vi "FOCUS_V42_H37.vi"(9 "X-pixels":sgl=256.0, 11 "Run":bool) -> (0 "Retrace pixels":sgl, 10 "Pixel Clock (Hz)":sgl)   [LabVIEW 2010] (continued)
      n95 = local write "ScanLineFScope"(sgl[][] [[0.026666667, 0.10555588, 0.18413667, 0.2620946, 0.33912018, 0.4149288, 0.48917702, 0.5616217, 0.6319491, 0.69988036, 0.7651882, 0.8275282, 0.88674605, 0.9425593, 0.9947472, 1.043162, 1.087492, 1.127687, 1.163523, 1.1948596, 1.2216425, 1.2436236, 1.2608614, 1.2732126, 1.2806307, 1.2831601, 1.280641, 1.2732344, 1.2608918, 1.2436653, 1.2216938, 1.1949208, 1.1635948, 1.1277666, 1.0875816, 1.0432596, 0.9948533, 0.9426741, 0.8868671, 0.8276569, 0.7653226, 0.70002097, 0.6320957, 0.5617722, 0.48933217, 0.41508698, 0.33928153, 0.2622585, 0.18430196, 0.10572225, 0.026833316, -0.052056268, -0.13063815, -0.20859744, -0.28562555, -0.36143658, -0.43568876, -0.50813806, -0.57846946, -0.6464066, -0.71171933, -0.77406645, -0.833292, -0.8891114, -0.941308, -0.9897297, -1.0340693, -1.0742743, -1.110118, -1.1414653, -1.1682563, -1.1902486, -1.2074977, -1.2198576, -1.2272873, -1.2298253, -1.2273177, -1.2199228, -1.2075888, -1.1903737, -1.1684103, -1.1416483, -1.110333, -1.0745125, -1.0343375, -0.99002266, -0.9416256, -0.8894551, -0.83365417, -0.7744517, -0.71212274, -0.6468276, -0.57890815, -0.5085887, -0.43615317, -0.36191097, -0.28610873, -0.20908824, -0.13062674, -0.05199747], [-1.2831608, -1.2806358, -1.2732235, -1.2608767, -1.2436445, -1.2216686, -1.1948903, -1.163559, -1.1277268, -1.0875369, -1.0432112, -0.9948003, -0.94261676, -0.88680667, -0.8275926, -0.7652557, -0.69995075, -0.6320225, -0.56169707, -0.48925468, -0.41500804, -0.33920097, -0.26217666, -0.18421942, -0.105639175, -0.026750105, 0.052139297, 0.13072063, 0.20867924, 0.28570607, 0.3615159, 0.4357661, 0.5082131, 0.57854253, 0.6464767, 0.71178705, 0.7741306, 0.83335227, 0.88916856, 0.9413609, 0.9897791, 1.034114, 1.0743139, 1.1101538, 1.1414957, 1.1682826, 1.1902695, 1.2075129, 1.2198684, 1.2272923, 1.2298261, 1.2273127, 1.2199119, 1.2075737, 1.1903529, 1.1683854, 1.1416179, 1.1102973, 1.0744729, 1.034293, 0.98997456, 0.94157284, 0.889398, 0.833594, 0.7743877, 0.7120561, 0.6467577, 0.5788353, 0.50851387, 0.4360761, 0.3618324, 0.28602856, 0.20900682, 0.13105093, 0.052471776, -0.026417017, -0.10530679, -0.18388921, -0.2618492, -0.33887854, -0.4146908, -0.48894495, -0.56139654, -0.63172984, -0.69966996, -0.76498514, -0.82733583, -0.8865652, -0.94238764, -0.9945887, -1.0430137, -1.0873581, -1.127568, -1.1634157, -1.1947683, -1.2215633, -1.2435613, -1.260816, -1.2693994, -1.2762786]] ("transposed array")) -> ()
    }
  }
  n96 = Type Cast(type="" ("name or relative path"), x=w48) -> (*(type *) &x=w45:string)
  n97 = Type Cast(type=tag "" ("6229 Device 2"), x=w65) -> (*(type *) &x=w64:tag)
  n98 = Type Cast(type=refnum<visa-resource-name> " " ("VISA Sutter MP-285"), x=w50) -> (*(type *) &x=w49:refnum<visa-resource-name>)
  n99 = Type Cast(type=refnum<visa-resource-name> refnum ("VISA Sutter MP-285"), x=w54) -> (*(type *) &x=w4:refnum<visa-resource-name>)
  n100 = property on="Run" class="Bool (strict)"("Visible"=w100) -> ()  [unwired: 2 in, 2 out]
  n101 = local write "End experiment"(w101) -> ()
  n102 = property on="colour table" class="Arr (strict)"("Value"=w37) -> ()  [unwired: 2 in, 2 out]
  n103 = property on="Galvos" class="XYGraph (strict)"("X Scale.Range:Minimum"=w3, "X Scale.Range:Maximum"="Scangraph scaling", "Y Scale.Range:Minimum"=w2, "Y Scale.Range:Maximum"="Scangraph scaling") -> ()  [unwired: 2 in, 2 out]
  n104 = Type Cast(type=u16 0 ("Program Version"), x=w84) -> (*(type *) &x=→"Program Version":u16)
  n105 = String To Path(string=w45) -> (path=w44:path)
  n106 = local write "FocusModeSelector"(TRUE ("FocusModeSelector")) -> ()
  n107 = local write "new FreeLine?"(FALSE ("new udl?")) -> ()
  n108 = local write "NewScanpattern"(FALSE ("NewScanpattern")) -> ()
  n109 = local write "VISA XPG-ADC"(w49) -> ()
  n110 = local write "AO/DIO Device"(w67) -> ()
  n111 = local write "VISA Sutter MP-285"(w4) -> ()
  n112 = property on="stop 2" class="Bool (strict)"("Visible"=w100) -> ()  [unwired: 2 in, 2 out]
  n113 = property on="Scan format" class="Ring (strict)"("Disabled"=u8 0) -> ()  [unwired: 2 in, 2 out]
  n114 = local write "AI Device"(w64) -> ()
  n115 = local write "MaiTai setting Path"(w44) -> ()
  n116 = local write "reset?"(125.0 ("reset?")) -> ()
  n117 = property on="Image 2" class="IntGraph (strict)"("Color Table"=w37) -> ()  [unwired: 2 in, 2 out]
  n118 = property on="End experiment" class="Bool (strict)"("Visible"=w100) -> ()  [unwired: 2 in, 2 out]
  n119 = local write "stop 2"(w101) -> ()
  n120 = property on="Hit Graph" class="IntGraph (strict)"("Color Table"=w37) -> ()  [unwired: 2 in, 2 out]
  n121 = while {
    tunnel: w6 -> [w207]
    tunnel: [w162] -> w5
    stop <- w163 stop-if-true
    n122 = flat-sequence {
      tunnel: [w1453] -> w295
      tunnel: w295 -> [w1668]
      tunnel: [w1626] -> w177
      tunnel: [w1641] -> w175
      tunnel: ["Zoom 1 scan voltage"] -> w174
      tunnel: [w1638] -> w173
      tunnel: [w1637] -> w172
      tunnel: [w1622] -> w170
      tunnel: [w1621] -> w169
      tunnel: [w2017] -> w259
      tunnel: [w2016] -> w288
      tunnel: [w1902] -> w290
      tunnel: [w2008] -> w260
      tunnel: [w1963] -> w298
      tunnel: [w1956] -> w262
      tunnel: [w1923] -> w297
      tunnel: [w2014] -> w261
      tunnel: [w2013] -> w285
      tunnel: [w2038] -> w283
      tunnel: [w2031] -> w282
      tunnel: w176 -> [w1887]
      tunnel: w186 -> [w1886]
      tunnel: [w1885] -> w182
      tunnel: w177 -> [w1873]
      tunnel: w175 -> [w1859]
      tunnel: w174 -> [w1872]
      tunnel: w173 -> [w1871]
      tunnel: w172 -> [w1870]
      tunnel: w171 -> [w1868]
      tunnel: w170 -> [w1864]
      tunnel: w169 -> [w1863]
      tunnel: [w1860] -> w168
      frame #0 {
        n123 = property on="Fiberscope" class="TabCtl (strict)"("Visible"="Fiberscope\nMode") -> ()  [unwired: 2 in, 2 out]
        n124 = property on="Hit Graph" class="IntGraph (strict)"("Visible"="Fiberscope\nMode") -> ()  [unwired: 2 in, 2 out]
        n125 = property on="Scale" class="Slide (strict)"("Visible"="Fiberscope\nMode") -> ()  [unwired: 2 in, 2 out]
        n126 = case shown="False" "Fiberscope\nMode" {
          tunnel: ["Mode selector" "Mode selectorFScope"] -> w1453
          frame False {
            n127 = case shown="0, Default" "Scan format" {
              tunnel: [w1559 sgl 64.0 ("X-pixels") sgl 128.0 ("X-pixels") sgl 256.0 ("X-pixels") sgl 512.0 ("X-pixels") sgl 32.0 ("X-pixels")] -> w1484
              tunnel: [w1558 sgl 64.0 ("Y-lines") sgl 128.0 ("Y-lines") sgl 256.0 ("Y-lines") sgl 512.0 ("Y-lines") sgl 32.0 ("Y-lines")] -> w1483
              tunnel: [w1557 sgl 2.0 ("line scan time (ms)") sgl 2.0 ("line scan time (ms)") sgl 2.0 ("line scan time (ms)") sgl 2.0 ("line scan time (ms)") sgl 1.0 ("line scan time (ms)")] -> w1482
              tunnel: [0 2 2 2 2 2] -> w1481
              frame 0, Default {
                n128 = local read "line scan time (ms)"() -> (w1557:sgl)
                n129 = local read "X-pixels"() -> (w1559:sgl)
                n130 = local read "Y-lines"() -> (w1558:sgl)
              }
              frame 1 {
              }
              frame 2 {
              }
              frame 3 {
              }
              frame 4 {
              }
              frame 5 {
              }
            }
            n131 = case shown="0, Default" "Mode selector" {
              tunnel: [2 0 2 2 0 2] -> w1465
              tunnel: [0 1 2 3 1 4] -> w1475
              tunnel: [w1496 w1506 0 w1527 w1537 w1547] -> w1471
              tunnel: w1481 -> [w1496 w1506 _ _ w1537 _]
              tunnel: [0 0 2 2 0 2] -> w1466
              tunnel: [w1501 w1511 u16 0 ("Scan format") u16 0 ("Scan format") w1542 u16 0 ("Scan format")] -> w1480
              tunnel: [TRUE ("Visible") FALSE ("Visible") FALSE ("Visible") FALSE ("Visible") FALSE ("Visible") FALSE ("Visible")] -> w1473
              tunnel: [u8 2 ("Disabled") u8 2 ("Disabled") u8 2 ("Disabled") u8 0 ("Disabled") u8 2 ("Disabled") u8 0 ("Disabled")] -> w1470
              tunnel: [2 2 2 2 2 0] -> w1461
              tunnel: [2 0 0 2 0 2] -> w1464
              tunnel: [w1496 w1506 2 w1527 w1537 w1547] -> w1463
              tunnel: [u8 2 ("Disabled") u8 2 ("Disabled") u8 0 ("Disabled") u8 0 ("Disabled") u8 2 ("Disabled") u8 2 ("Disabled")] -> w1462
              frame 0, Default {
                # "Focus mode"
                n132 = local read "Scan format"() -> (w1501:u16)
              }
              frame 1 {
                # "frame scan"
                n133 = local read "Scan format"() -> (w1511:u16)
              }
              frame 2 {
                # "straight line scan"
              }
              frame 3 {
                w1527 = 2
                # "user-defined line"
              }
              frame 4 {
                # "frame scan piezo"
                n134 = local read "Scan format"() -> (w1542:u16)
              }
              frame 5 {
                w1547 = 2
                # "user-defined line 3D"
              }
            }
            "frame/line indicator" <- w1475
            n135 = Less?(x=w1475, y=u16 3) -> (x < y?=w1477:bool)
            n136 = case shown="False" w1477 {
              tunnel: [TRUE ("Visible") FALSE ("Visible")] -> w1476
              tunnel: [w1488 FALSE ("Visible")] -> w1472
              frame False {
                n137 = property on="Image 3" class="IntGraph (strict)"() -> ("Visible"=w1488:bool)  [unwired: 2 in, 2 out]
              }
              frame True {
              }
            }
            n138 = case shown="3" "Scan format 2" {
              tunnel: [i16 10 ("X-pixels") i16 20 ("X-pixels") i16 40 ("X-pixels") i16 60 ("X-pixels")] -> w1468
              frame 0, Default {
              }
              frame 1 {
              }
              frame 2 {
              }
              frame 3 {
              }
            }
            n139 = local write "X-pixels"(w1484) -> ()
            n140 = local write "Y-lines"(w1483) -> ()
            n141 = local write "line scan time (ms)"(w1482) -> ()
            n142 = property on="phase shift [°]" class="DigNum (strict)"("Disabled"=w1461) -> ()  [unwired: 2 in, 2 out]
            n143 = local write "Scan format"(w1480) -> ()
            n144 = property on="Number of frames" class="DigNum (strict)"("Disabled"=w1464) -> ()  [unwired: 2 in, 2 out]
            n145 = property on="Averaging" class="DigNum (strict)"("Disabled"=w1465) -> ()  [unwired: 2 in, 2 out]
            n146 = property on="z-step (um)" class="DigNum (strict)"("Disabled"=w1465) -> ()  [unwired: 2 in, 2 out]
            n147 = property on="Scan format" class="Ring (strict)"("Disabled"=w1466) -> ()  [unwired: 2 in, 2 out]
            n148 = property on="X-pixels" class="DigNum (strict)"("Disabled"=w1471) -> ()  [unwired: 2 in, 2 out]
            n149 = property on="#" class="DigNum (strict)"("Disabled"=w1471) -> ()  [unwired: 2 in, 2 out]
            n150 = property on="line scan time (ms)" class="DigNum (strict)"("Disabled"=w1471) -> ()  [unwired: 2 in, 2 out]
            n151 = property on="#" class="DigNum (strict)"("Disabled"=w1470) -> ()  [unwired: 2 in, 2 out]
            n152 = property on="Y-lines FreeLine" class="DigNum (strict)"("Disabled"=w1470) -> ()  [unwired: 2 in, 2 out]
            n153 = property on="Y-Scale" class="Bool (strict)"("Disabled"=w1462) -> ()  [unwired: 2 in, 2 out]
            n154 = local write "ImageSelector"(w1472) -> ()
            n155 = property on="XY Graph 1" class="XYGraph (strict)"("Visible"=w1476) -> ()  [unwired: 2 in, 2 out]
            n156 = property on="XY Graph 2" class="XYGraph (strict)"("Visible"=w1476) -> ()  [unwired: 2 in, 2 out]
            n157 = property on="Image 3" class="IntGraph (strict)"("Visible"=w1472) -> ()  [unwired: 2 in, 2 out]
            n158 = property on="Histogram1" class="XYGraph (strict)"("Visible"=w1472) -> ()  [unwired: 2 in, 2 out]
            n159 = property on="Y-lines" class="DigNum (strict)"("Disabled"=w1463) -> ()  [unwired: 2 in, 2 out]
            n160 = Divide(x=4000.0, y=w1468) -> (x/y=→"pixelstoµm":dbl)
            n161 = property on="FocusModeSelector" class="Bool (strict)"("Visible"=w1473) -> ()  [unwired: 2 in, 2 out]
            n162 = property on="XY Graph 3" class="XYGraph (strict)"("Visible"=FALSE) -> ()  [unwired: 2 in, 2 out]
            n163 = property on="XY Graph 4" class="XYGraph (strict)"("Visible"=w1476) -> ()  [unwired: 2 in, 2 out]
            n164 = property on="Image 4" class="IntGraph (strict)"("Visible"=w1472) -> ()  [unwired: 2 in, 2 out]
            n165 = property on="Amplitude Factor" class="DigNum (strict)"("Disabled"=w1461) -> ()  [unwired: 2 in, 2 out]
            n166 = property on="z frequency" class="Slide (strict)"("Disabled"=w1461) -> ()  [unwired: 2 in, 2 out]
            n167 = property on="Histogram2" class="XYGraph (strict)"("Visible"=w1472) -> ()  [unwired: 2 in, 2 out]
            n168 = local write "Open?"(FALSE ("Open?")) -> ()
            n169 = property on="new FreeLine?" class="Bool (strict)"("Disabled"=w1470) -> ()  [unwired: 2 in, 2 out]
            n170 = property on="#" class="DigNum (strict)"("Disabled"=w1464) -> ()  [unwired: 2 in, 2 out]
            n171 = property on="#" class="DigNum (strict)"("Disabled"=w1465) -> ()  [unwired: 2 in, 2 out]
            n172 = property on="Time interval [s]" class="DigNum (strict)"("Disabled"=w1465) -> ()  [unwired: 2 in, 2 out]
            n173 = property on="Number of stacks" class="DigNum (strict)"("Disabled"=w1465) -> ()  [unwired: 2 in, 2 out]
            n174 = property on="#" class="DigNum (strict)"("Disabled"=w1465) -> ()  [unwired: 2 in, 2 out]
            n175 = property on="Cusp Delay" class="DigNum (strict)"("Disabled"=w1466) -> ()  [unwired: 2 in, 2 out]
          }
          frame True {
            n176 = local write "Mode selector"("Mode selectorFScope") -> ()
            n177 = case shown="0, Default" "Mode selectorFScope" {
              tunnel: [u16 2 ("Mode selectorFScope") u16 0 ("Mode selectorFScope") u16 2 ("Mode selectorFScope")] -> w1580
              tunnel: [u16 0 ("Mode selectorFScope") u16 0 ("Mode selectorFScope") u16 2 ("Mode selectorFScope")] -> w1583
              tunnel: [w1594 w1597 u16 0 ("Scan format FScope")] -> w1582
              frame 0, Default {
                n178 = local read "Scan format FScope"() -> (w1594:u16)
              }
              frame 1 {
                n179 = local read "Scan format FScope"() -> (w1597:u16)
              }
              frame 2 {
              }
            }
            n180 = local write "frame/line indicator"("Mode selectorFScope") -> ()
            n181 = local write "Time interval [s]"("Time interval [s]") -> ()
            n182 = local write "Number of stacks"("Number of Stacks") -> ()
            n183 = local read "Number of Frames"() -> (w1589:sgl)
            n184 = case shown="0, Default" "Scan format FScope" {
              tunnel: [w1605 sgl 64.0 ("X dim") sgl 128.0 ("X dim") sgl 256.0 ("X dim") sgl 512.0 ("X dim") sgl 32.0 ("X dim")] -> w1591
              tunnel: [w1604 sgl 64.0 ("Y dim") sgl 128.0 ("Y dim") sgl 256.0 ("Y dim") sgl 512.0 ("Y dim") sgl 32.0 ("Y dim")] -> w1590
              tunnel: [u8 0 ("Disabled") u8 2 ("Disabled") u8 2 ("Disabled") u8 2 ("Disabled") u8 2 ("Disabled") u8 2 ("Disabled")] -> w1592
              frame 0, Default {
                n185 = local read "Y dim"() -> (w1604:sgl)
                n186 = local read "X dim"() -> (w1605:sgl)
              }
              frame 1 {
              }
              frame 2 {
              }
              frame 3 {
              }
              frame 4 {
              }
              frame 5 {
              }
            }
            n187 = local read "Averaging"() -> (w1588:sgl)
            n188 = local write "Scan format FScope"(w1582) -> ()
            n189 = property on="Scan format FScope" class="Ring (strict)"("Disabled"=w1583) -> ()  [unwired: 2 in, 2 out]
            n190 = property on="Time interval [s]" class="DigNum (strict)"("Disabled"=w1580) -> ()  [unwired: 2 in, 2 out]
            n191 = property on="Number of Stacks" class="DigNum (strict)"("Disabled"=w1580) -> ()  [unwired: 2 in, 2 out]
            n192 = property on="Number of Frames" class="DigNum (strict)"("Disabled"=w1580) -> ()  [unwired: 2 in, 2 out]
            n193 = property on="Averaging" class="DigNum (strict)"("Disabled"=w1580) -> ()  [unwired: 2 in, 2 out]
            n194 = property on="#" class="DigNum (strict)"("Disabled"=w1580) -> ()  [unwired: 2 in, 2 out]
            n195 = property on="#" class="DigNum (strict)"("Disabled"=w1580) -> ()  [unwired: 2 in, 2 out]
            n196 = property on="#" class="DigNum (strict)"("Disabled"=w1580) -> ()  [unwired: 2 in, 2 out]
            n197 = local write "X dim"(w1591) -> ()
            n198 = local write "Y dim"(w1590) -> ()
            n199 = property on="Y dim" class="DigNum (strict)"("Disabled"=w1592) -> ()  [unwired: 2 in, 2 out]
            n200 = local write "Number of frames"(w1589) -> ()
            n201 = local write "Averaging"(w1588) -> ()
            n202 = global write "GlobelFSCOPE.vi" "X dim"(w1591) -> ()
            n203 = global write "GlobelFSCOPE.vi" "Y dim"(w1590) -> ()
            n204 = property on="X dim" class="DigNum (strict)"("Disabled"=w1592) -> ()  [unwired: 2 in, 2 out]
            n205 = local write "X-pixels"("X dim") -> ()
            n206 = local write "Y-lines"("Y dim") -> ()
            n207 = global write "GlobelFSCOPE.vi" "Y dim"("Y dim") -> ()
            n208 = global write "GlobelFSCOPE.vi" "X dim"("X dim") -> ()
          }
        }
        n209 = local read "GetFirst"() -> (w1447:bool)
        n210 = local read "GetLast"() -> (w1446:bool)
        n211 = And(x=w1447, y=w1446) -> (x .and. y?=w1445:bool)
        n212 = case shown="True" w1445 {
          frame False {
          }
          frame True {
            n213 = local read "Number of frames"() -> (w1457:sgl)
            n214 = local read "FirstPosition"() -> (w1454:sgl)
            n215 = local read "LastPosition"() -> (w1455:sgl)
            n216 = Decrement(x=w1457) -> (x-1=w1458:sgl)
            n217 = Subtract(x=w1455, y=w1454) -> (x-y=w1459:sgl)
            n218 = Divide(x=w1459, y=w1458) -> (x/y=w1456:sgl)
            n219 = local write "z-step (um)"(w1456) -> ()
          }
        }
        n220 = Get Date/Time String(date format (0)=enum16{"short", "long", "abbreviated"}."abbreviated") -> (time string=→"Time":string)  [unwired: 2 in, 1 out]
        n221 = Format Date/Time String(time format string (%c)="%m%d%y") -> (date/time string=→"Date":string)  [unwired: 2 in]
      }
      frame #1 {
        # "Line scan position and measurement cursors"
        n222 = local read "frame/line indicator"() -> (w1641:u16)
        n223 = Less?(x=w1668, y=3.0) -> (x < y?=w1663:bool)
        n224 = And(x="View line\ncheck box", y=w1663) -> (x .and. y?=w1667:bool)
        n225 = And(x=w1663, y="Measurement cursor check box") -> (x .and. y?=w1662:bool)
        n226 = control-ref of="Image 2"() -> (w1665:refnum<vi>)
        n227 = control-ref of="Image 1"() -> (w1666:refnum<vi>)
        n228 = Divide(x="Y-lines", y="X-pixels") -> (x/y=w1671:sgl)
        n229 = case "Measurement cursor on/off" shown="True" w1662 {
          tunnel: w1665 -> [w1745 w1751]
          tunnel: w1666 -> [w1746 w1752]
          frame False {
            w1744 = FALSE ("Cursor.Visible")
            w1747 = u32 1 ("Active Cursor")
            n230 = property on="OGB value" class="DigNum (strict)"("Visible"=w1744) -> ()  [unwired: 2 in, 2 out]
            n231 = property on="Alexa value" class="DigNum (strict)"("Visible"=w1744) -> ()  [unwired: 2 in, 2 out]
            n232 = property on="Property Node" class="IntGraph (strict)"(reference=w1746, "Active Cursor"=w1747, "Cursor.Visible"=w1744) -> ()  [unwired: 1 in, 2 out]
            n233 = property on="Property Node" class="IntGraph (strict)"(reference=w1745, "Active Cursor"=w1747, "Cursor.Visible"=w1744) -> ()  [unwired: 1 in, 2 out]
          }
          frame True {
            w1748 = u32 1 ("Active Cursor")
            w1753 = u32 16776960
            w1749 = TRUE ("Cursor.Visible")
            w1754 = u32 1 ("Active Cursor")
            n234 = while {
              tunnel: w1752 -> [w1765]
              tunnel: w1751 -> [w1764]
              stop <- w1755 continue-if-true
              w1763 = u32 1 ("Active Cursor")
              n235 = property on="Property Node" class="IntGraph (strict)"(reference=w1765, "Active Cursor"=w1763) -> ("Cursor.Cursor Position:Cursor X"=w1759:dbl, "Cursor.Cursor Position:Cursor Y"=w1757:dbl, "Value"=w1762:u8[][])  [unwired: 1 in, 2 out]
              n236 = Index Array(array=w1762, index (row)=w1759, index (col)=w1757) -> (element=→"OGB value":u8)
              n237 = property on="Property Node" class="IntGraph (strict)"(reference=w1764, "Active Cursor"=w1763, "Cursor.Cursor Position:Cursor X"=w1759, "Cursor.Cursor Position:Cursor Y"=w1757) -> ("Value"=w1758:u8[][])  [unwired: 1 in, 2 out]
              n238 = Index Array(array=w1758, index (row)=w1759, index (col)=w1757) -> (element=→"Alexa value":u8)
              n239 = local read "Measurement cursor check box"() -> (w1756:bool)
              n240 = case shown="False" w1756 {
                selector: w1756 -> [w1766 w1768]
                tunnel: [w1766 w1768] -> w1755
                frame False {
                  n241 = property on="Run" class="Bool (strict)"("Disabled"=u8 0) -> ()  [unwired: 2 in, 2 out]
                }
                frame True {
                }
              }
            }
            n242 = property on="Run" class="Bool (strict)"("Disabled"=u8 2) -> ()  [unwired: 2 in, 2 out]
            n243 = property on="Property Node" class="IntGraph (strict)"(reference=w1752, "Active Cursor"=w1754, "Cursor.Visible"=w1749, "Cursor.Cursor Color"=w1753, "Cursor.Cursor Position:Cursor X"=w1748, "Cursor.Cursor Position:Cursor Y"=w1748) -> ()  [unwired: 1 in, 2 out]
            n244 = property on="Property Node" class="IntGraph (strict)"(reference=w1751, "Active Cursor"=w1754, "Cursor.Visible"=w1749, "Cursor.Cursor Color"=w1753) -> ()  [unwired: 1 in, 2 out]
            n245 = property on="OGB value" class="DigNum (strict)"("Visible"=w1749) -> ()  [unwired: 2 in, 2 out]
            n246 = property on="Alexa value" class="DigNum (strict)"("Visible"=w1749) -> ()  [unwired: 2 in, 2 out]
          }
        }
        n247 = Greater?(x=w1671, y=1.0) -> (0:w1672:bool)
        n248 = local read "Fiberscope\nMode"() -> (w1646:bool)
        n249 = case shown="True" w1646 {
          tunnel: [w1685 w1686] -> w1660
          frame False {
            n250 = local read "Mode selector"() -> (w1685:u16)
          }
          frame True {
            n251 = local read "Mode selectorFScope"() -> (w1686:u16)
          }
        }
        n252 = case shown="False" w1672 {
          tunnel: w1671 -> [w1775 _]
          tunnel: [w1774 w1814] -> w1654
          tunnel: [w1772 w1813] -> w1653
          tunnel: [w1771 w1812] -> w1652
          frame False {
            w1770 = u32 512 ("Plot Area:Size:Width")
            n253 = Multiply(x=w1770, y=w1775) -> (x*y=w1769:sgl)
            n254 = property on="Image 1" class="IntGraph (strict)"("Plot Area:Size:Width"=w1770, "Plot Area:Size:Height"=w1769) -> ()  [unwired: 2 in, 2 out]
            n255 = property on="Image 2" class="IntGraph (strict)"("Plot Area:Size:Width"=w1770, "Plot Area:Size:Height"=w1769) -> ()  [unwired: 2 in, 2 out]
            n256 = property on="ImageSlide" class="Slide (strict)"("Housing Size:Height"=w1769) -> ()  [unwired: 2 in, 2 out]
            n257 = property on="XY Graph 1" class="XYGraph (strict)"("Plot Area:Size:Width"=w1770, "Plot Area:Size:Height"=w1769) -> ()  [unwired: 2 in, 2 out]
            n258 = property on="XY Graph 2" class="XYGraph (strict)"("Plot Area:Size:Width"=w1770, "Plot Area:Size:Height"=w1769) -> ()  [unwired: 2 in, 2 out]
            n259 = property on="SlideHorizontal" class="Slide (strict)"("Housing Size:Width"=w1770) -> ()  [unwired: 2 in, 2 out]
            n260 = property on="XY Graph 3" class="XYGraph (strict)"("Plot Area:Size:Width"=w1770, "Plot Area:Size:Height"=w1769) -> ()  [unwired: 2 in, 2 out]
            n261 = property on="XY Graph 4" class="XYGraph (strict)"("Plot Area:Size:Width"=w1770, "Plot Area:Size:Height"=w1769) -> ()  [unwired: 2 in, 2 out]
            n262 = local read "frame/line indicator"() -> (w1773:u16)
            n263 = case shown="2" w1773 {
              tunnel: [FALSE ("Visible") w1782 w1792 w1796 w1805] -> w1774
              tunnel: [_ w1780 w1789 w1797 w1803] -> w1772
              tunnel: [FALSE ("Visible") FALSE ("Visible") FALSE ("Visible") FALSE ("Visible") TRUE ("Visible")] -> w1771
              frame 0, Default {
              }
              frame 1 {
                n264 = local read "Number of frames"() -> (w1779:sgl)
                n265 = Decrement(x=w1779) -> (x-1=w1780:sgl)
                n266 = Less Or Equal To 0?(x=w1780) -> (x <= 0?=w1781:bool)
                n267 = case shown="False" w1781 {
                  tunnel: [TRUE ("Visible") FALSE ("Visible")] -> w1782
                  frame False {
                  }
                  frame True {
                  }
                }
              }
              frame 2 {
                n268 = local read "Y-lines"() -> (w1787:sgl)
                n269 = local read "Number of frames"() -> (w1785:sgl)
                n270 = Multiply(x=w1787, y=w1785) -> (x*y=w1786:sgl)
                n271 = local read "X-pixels"() -> (w1791:sgl)
                n272 = Subtract(x=w1786, y=w1791) -> (x-y=w1789:sgl)
                n273 = Less Or Equal To 0?(x=w1789) -> (x <= 0?=w1790:bool)
                n274 = case shown="False" w1790 {
                  tunnel: [TRUE ("Visible") FALSE ("Visible")] -> w1792
                  frame False {
                  }
                  frame True {
                  }
                }
              }
              frame 3 {
                n275 = local read "X-pixels FreeLine"() -> (w1799:sgl)
                n276 = local read "Y-lines FreeLine"() -> (w1800:sgl)
                n277 = Subtract(x=w1800, y=w1799) -> (x-y=w1797:sgl)
                n278 = Less Or Equal To 0?(x=w1797) -> (x <= 0?=w1798:bool)
                n279 = case shown="True" w1798 {
                  tunnel: [TRUE ("Visible") FALSE ("Visible")] -> w1796
                  frame False {
                  }
                  frame True {
                  }
                }
              }
              frame 4 {
                n280 = local read "X-pixels FreeLine"() -> (w1807:sgl)
                n281 = local read "Y-lines FreeLine"() -> (w1808:sgl)
                n282 = Subtract(x=w1808, y=w1807) -> (x-y=w1803:sgl)
                n283 = Less Or Equal To 0?(x=w1803) -> (x <= 0?=w1806:bool)
                n284 = case shown="True" w1806 {
                  tunnel: [FALSE ("Visible") FALSE ("Visible")] -> w1805
                  frame False {
                  }
                  frame True {
                  }
                }
              }
            }
          }
          frame True {
            w1811 = 512
            n285 = property on="Image 1" class="IntGraph (strict)"("Plot Area:Size:Width"=w1811, "Plot Area:Size:Height"=w1811) -> ()  [unwired: 2 in, 2 out]
            n286 = property on="Image 2" class="IntGraph (strict)"("Plot Area:Size:Width"=w1811, "Plot Area:Size:Height"=w1811) -> ()  [unwired: 2 in, 2 out]
            n287 = property on="ImageSlide" class="Slide (strict)"("Housing Size:Height"=w1811) -> ()  [unwired: 2 in, 2 out]
            n288 = property on="XY Graph 1" class="XYGraph (strict)"("Plot Area:Size:Width"=w1811, "Plot Area:Size:Height"=w1811) -> ()  [unwired: 2 in, 2 out]
            n289 = property on="XY Graph 2" class="XYGraph (strict)"("Plot Area:Size:Width"=w1811, "Plot Area:Size:Height"=w1811) -> ()  [unwired: 2 in, 2 out]
            n290 = property on="SlideHorizontal" class="Slide (strict)"("Housing Size:Width"=w1811) -> ()  [unwired: 2 in, 2 out]
            n291 = local read "frame/line indicator"() -> (w1815:u16)
            n292 = property on="XY Graph 4" class="XYGraph (strict)"("Plot Area:Size:Width"=w1811, "Plot Area:Size:Height"=w1811) -> ()  [unwired: 2 in, 2 out]
            n293 = property on="XY Graph 3" class="XYGraph (strict)"("Plot Area:Size:Width"=w1811, "Plot Area:Size:Height"=w1811) -> ()  [unwired: 2 in, 2 out]
            n294 = case shown="2" w1815 {
              tunnel: [FALSE ("Visible") w1821 w1831 w1838 w1846] -> w1814
              tunnel: [_ w1822 w1832 w1837 w1845] -> w1813
              tunnel: [FALSE ("Visible") FALSE ("Visible") FALSE ("Visible") FALSE ("Visible") TRUE ("Visible")] -> w1812
              frame 0, Default {
                n295 = One Button Dialog(message="Unable to display the whole image using these settings.\nThe requested image can be acquired and saved, but\n      the displayed image will be clipped.\nThis is because the y-dimension (# lines) is larger\n      than the x-dimension (# pixels).\nTo solve this problem, switch the values of x- and y-\n      dimensions (and rotate the image, if necessary).") -> ()  [unwired: 1 in, 1 out]
              }
              frame 1 {
                n296 = local read "Number of frames"() -> (w1820:sgl)
                n297 = Decrement(x=w1820) -> (x-1=w1822:sgl)
                n298 = Less Or Equal To 0?(x=w1822) -> (x <= 0?=w1823:bool)
                n299 = case shown="False" w1823 {
                  tunnel: [TRUE ("Visible") FALSE ("Visible")] -> w1821
                  frame False {
                  }
                  frame True {
                  }
                }
              }
              frame 2 {
                n300 = local read "Y-lines"() -> (w1828:sgl)
                n301 = local read "Number of frames"() -> (w1827:sgl)
                n302 = local read "X-pixels"() -> (w1830:sgl)
                n303 = Multiply(x=w1828, y=w1827) -> (x*y=w1826:sgl)
                n304 = Subtract(x=w1826, y=w1830) -> (x-y=w1832:sgl)
                n305 = Less Or Equal To 0?(x=w1832) -> (x <= 0?=w1833:bool)
                n306 = case shown="False" w1833 {
                  tunnel: [TRUE ("Visible") FALSE ("Visible")] -> w1831
                  frame False {
                  }
                  frame True {
                  }
                }
              }
              frame 3 {
                n307 = local read "X-pixels FreeLine"() -> (w1840:sgl)
                n308 = local read "Y-lines FreeLine"() -> (w1841:sgl)
                n309 = Subtract(x=w1841, y=w1840) -> (x-y=w1837:sgl)
                n310 = Less Or Equal To 0?(x=w1837) -> (x <= 0?=w1839:bool)
                n311 = case shown="False" w1839 {
                  tunnel: [TRUE ("Visible") FALSE ("Visible")] -> w1838
                  frame False {
                  }
                  frame True {
                  }
                }
              }
              frame 4 {
                n312 = local read "X-pixels FreeLine"() -> (w1848:sgl)
                n313 = local read "Y-lines FreeLine"() -> (w1849:sgl)
                n314 = Subtract(x=w1849, y=w1848) -> (x-y=w1845:sgl)
                n315 = Less Or Equal To 0?(x=w1845) -> (x <= 0?=w1847:bool)
                n316 = case shown="False" w1847 {
                  tunnel: [FALSE ("Visible") FALSE ("Visible")] -> w1846
                  frame False {
                  }
                  frame True {
                  }
                }
              }
            }
          }
        }
        "ImageSlideMax" <- w1653
        n317 = Bundle("frame/line indicator"=w1641, "X-pixels"="X-pixels", "Y-lines"="Y-lines", "line scan time (ms)"="line scan time (ms)", "Zoom 1 scan voltage"="Zoom 1 scan voltage", "Scanblock Factor"="Scanblock Factor", "Scanpattern"="Scanpattern") -> (w1636:T13)  [unwired: 1 in]
        n318 = case "Cursors to indicate line scan position" shown="True" w1667 {
          tunnel: w1666 -> [w1732 w1736]
          tunnel: w1665 -> [w1731 w1735]
          frame False {
            w1733 = FALSE ("Cursor.Visible")
            w1734 = u32 0 ("Active Cursor")
            n319 = property on="Property Node" class="IntGraph (strict)"(reference=w1732, "Active Cursor"=w1734, "Cursor.Visible"=w1733) -> ()  [unwired: 1 in, 2 out]
            n320 = property on="Property Node" class="IntGraph (strict)"(reference=w1731, "Active Cursor"=w1734, "Cursor.Visible"=w1733) -> ()  [unwired: 1 in, 2 out]
          }
          frame True {
            w1740 = u32 14418136
            w1743 = TRUE ("Cursor.Visible")
            w1742 = -1.0 ("Cursor.Cursor Position:Cursor X")
            w1741 = u32 0 ("Active Cursor")
            n321 = local read "Y-lines"() -> (w1737:sgl)
            n322 = Divide(x=w1737, y=2.0) -> (x/y=w1738:dbl)
            n323 = property on="Property Node" class="IntGraph (strict)"(reference=w1736, "Active Cursor"=w1741, "Cursor.Cursor Position:Cursor X"=w1742, "Cursor.Cursor Position:Cursor Y"=w1738, "Cursor.Visible"=w1743, "Cursor.Cursor Color"=w1740) -> ()  [unwired: 1 in, 2 out]
            n324 = property on="Property Node" class="IntGraph (strict)"(reference=w1735, "Active Cursor"=w1741, "Cursor.Cursor Position:Cursor X"=w1742, "Cursor.Cursor Position:Cursor Y"=w1738, "Cursor.Visible"=w1743, "Cursor.Cursor Color"=w1740) -> ()  [unwired: 1 in, 2 out]
          }
        }
        n325 = case shown="2" w1660 {
          tunnel: "X-pixels" -> [w1687 w1710 w1713 w1730]
          tunnel: "Y-lines" -> [w1688 w1709 _ w1729]
          tunnel: "X-pixels" -> [w1698 w1708 w1714 w1728]
          tunnel: "Y-lines" -> [w1697 w1707 _ w1727]
          tunnel: [0.0 ("X Scale.Range:Minimum") 0.0 ("X Scale.Range:Minimum") 0.0 ("X Scale.Range:Minimum") 0.0 ("X Scale.Range:Minimum")] -> w1650
          tunnel: [w1695 w1705 w1712 w1725] -> w1649
          tunnel: [0.0 ("Y Scale.Range:Minimum") 0.0 ("Y Scale.Range:Minimum") 0.0 ("Y Scale.Range:Minimum") 0.0 ("Y Scale.Range:Minimum")] -> w1648
          tunnel: [w1693 w1703 w1712 w1723] -> w1647
          tunnel: [0.0 ("X Scale.Range:Minimum") 0.0 ("X Scale.Range:Minimum") 0.0 ("X Scale.Range:Minimum") 0.0 ("X Scale.Range:Minimum")] -> w1659
          tunnel: [w1691 w1701 w1711 w1721] -> w1658
          tunnel: [0.0 ("Y Scale.Range:Minimum") 0.0 ("Y Scale.Range:Minimum") 0.0 ("Y Scale.Range:Minimum") 0.0 ("Y Scale.Range:Minimum")] -> w1657
          tunnel: [w1689 w1699 w1711 w1719] -> w1655
          frame 0, Default {
            n326 = Decrement(x=w1687) -> (x-1=w1695:sgl)
            n327 = Decrement(x=w1688) -> (x-1=w1693:sgl)
            n328 = Decrement(x=w1698) -> (x-1=w1691:sgl)
            n329 = Decrement(x=w1697) -> (x-1=w1689:sgl)
          }
          frame 1 {
            n330 = Decrement(x=w1710) -> (x-1=w1705:sgl)
            n331 = Decrement(x=w1709) -> (x-1=w1703:sgl)
            n332 = Decrement(x=w1708) -> (x-1=w1701:sgl)
            n333 = Decrement(x=w1707) -> (x-1=w1699:sgl)
          }
          frame 2 {
            n334 = Decrement(x=w1713) -> (x-1=w1712:sgl)
            n335 = Decrement(x=w1714) -> (x-1=w1711:sgl)
          }
          frame 4 {
            n336 = Decrement(x=w1730) -> (x-1=w1725:sgl)
            n337 = Decrement(x=w1729) -> (x-1=w1723:sgl)
            n338 = Decrement(x=w1728) -> (x-1=w1721:sgl)
            n339 = Decrement(x=w1727) -> (x-1=w1719:sgl)
          }
        }
        n340 = case shown="True" "Scanpattern" {
          tunnel: [w1679 w1684] -> w1643
          tunnel: [w1678 w1683] -> w1638
          tunnel: [w1677 w1682] -> w1637
          tunnel: w1636 -> [w1676 w1681]
          tunnel: [w1675 w1680] -> w1622
          frame True {
            n341 = call "ScanGeniFOCUS.vi"("Parameters In"=w1676) -> ("X-Scansignals"=w1678:dbl[], "Parameters out"=w1679:T14, "Y-Scansignals"=w1677:dbl[], "Z-Scansignals"=w1675:dbl[])
          }
          frame False {
            n342 = call "ScanGeniFOCUS.vi"("Parameters In"=w1681) -> ("X-Scansignals"=w1683:dbl[], "Parameters out"=w1684:T14, "Y-Scansignals"=w1682:dbl[], "Z-Scansignals"=w1680:dbl[])
          }
        }
        n343 = Unbundle(w1643) -> ("Scan mode"=w1623:u16, "Pixel Clock (Hz)"=→"Pixel Clock (Hz)":sgl, "pixel dwell time [us]"=w1626:sgl, "Frame rate (Hz)"=→"Frame rate [Hz]":sgl, "total x pixels"=→"total x pixels":sgl, "total y lines"=→"total y pixels":sgl, "Retrace pixels (tdown)"=→"Retrace pixels":sgl, "Scan Cut-Off (either end)"=→"Scan Cut-Off (either end)":sgl, "pixels in frame"=→"pixels in frame":sgl, "pixels in frame + yretrace"=→"pixels in frame + yretrace":sgl, "Scanblock length"=→"Scan Block Length":sgl, "total pixels in frame"=→"total pixels in frame":sgl, "Z-scan mode"=w1621:u16)
        "pixel dwell time [us]" <- w1626
        "Scan mode" <- w1623
        n344 = property on="Image 1" class="IntGraph (strict)"("X Scale.Range:Minimum"=w1650, "X Scale.Range:Maximum"=w1649, "Y Scale.Range:Minimum"=w1648, "Y Scale.Range:Maximum"=w1647) -> ()  [unwired: 2 in, 2 out]
        n345 = property on="Image 2" class="IntGraph (strict)"("X Scale.Range:Minimum"=w1659, "X Scale.Range:Maximum"=w1658, "Y Scale.Range:Minimum"=w1657, "Y Scale.Range:Maximum"=w1655) -> ()  [unwired: 2 in, 2 out]
        n346 = property on="Hit Graph" class="IntGraph (strict)"("X Scale.Range:Minimum"=w1650, "X Scale.Range:Maximum"=w1649, "Y Scale.Range:Minimum"=w1648, "Y Scale.Range:Maximum"=w1647) -> ()  [unwired: 2 in, 2 out]
        n347 = case shown="0, Default" w1623 {
          frame 1 {
            n348 = property on="Shift" class="DigNum (strict)"("Visible"=TRUE) -> ()  [unwired: 2 in, 2 out]
          }
          frame 0, Default {
            n349 = property on="Shift" class="DigNum (strict)"("Visible"=FALSE) -> ()  [unwired: 2 in, 2 out]
          }
        }
        n350 = Not(x=w1652) -> (.not. x?=w1651:bool)
        n351 = local write "XScale"(w1651) -> ()
        n352 = property on="SlideHorizontal" class="Slide (strict)"("Visible"=w1652) -> ()  [unwired: 2 in, 2 out]
        n353 = property on="ImageSlide" class="Slide (strict)"("Scale.Range:Minimum"=0.0, "Scale.Range:Maximum"=w1653) -> ()  [unwired: 2 in, 2 out]
        n354 = property on="ImageSlide" class="Slide (strict)"("Visible"=w1654) -> ()  [unwired: 2 in, 2 out]
        n355 = property on="Play Movie" class="Bool (strict)"("Visible"=w1654) -> ()  [unwired: 2 in, 2 out]
        n356 = property on="Velocity" class="Slide (strict)"("Visible"=w1654) -> ()  [unwired: 2 in, 2 out]
      }
      frame #2 {
        w1959 = 10123 items=["Finite Samples"=10178, "Continuous Samples"=10123, "Hardware Timed Single Point"=12522] ("sample mode")
        w2012 = 10123 items=["Finite Samples"=10178, "Continuous Samples"=10123, "Hardware Timed Single Point"=12522] ("sample mode")
        w2020 = 10123 items=["Finite Samples"=10178, "Continuous Samples"=10123, "Hardware Timed Single Point"=12522] ("sample mode")
        w2034 = 2.0 ("Y Scale.Range:Maximum")
        w2035 = 1.0 ("Y Scale.Range:Minimum")
        w2036 = 0.0 ("X Scale.Range:Minimum")
        # "x-y plot of galvo signals"
        n357 = local read "frame/line indicator"() -> (w2029:u16)
        n358 = case shown="4" w2029 {
          tunnel: [w2988 w2989 w2991 w2993 w3005] -> w2033
          tunnel: [w2987 w2990 w2992 w2993 w2997] -> w2032
          frame 0, Default {
            n359 = property on="Image 3" class="IntGraph (strict)"() -> ("X Scale.Range:Maximum"=w2988:dbl, "Y Scale.Range:Maximum"=w2987:dbl)  [unwired: 2 in, 2 out]
          }
          frame 1 {
            n360 = property on="Image 3" class="IntGraph (strict)"() -> ("X Scale.Range:Maximum"=w2989:dbl, "Y Scale.Range:Maximum"=w2990:dbl)  [unwired: 2 in, 2 out]
          }
          frame 2 {
            n361 = property on="Image 3" class="IntGraph (strict)"() -> ("X Scale.Range:Maximum"=w2991:dbl, "Y Scale.Range:Maximum"=w2992:dbl)  [unwired: 2 in, 2 out]
          }
          frame 3 {
            n362 = local read "X-pixels FreeLine"() -> (w2994:sgl)
            n363 = Decrement(x=w2994) -> (x-1=w2993:sgl)
          }
          frame 4 {
            w3000 = sgl 1000000.0 ("y")
            n364 = local read "XScale"() -> (w3004:bool)
            n365 = local read "X-pixels FreeLine"() -> (w2995:sgl)
            n366 = case shown="True" w3004 {
              tunnel: [w3010 w3014] -> w3005
              tunnel: [w3010 w3013] -> w2996
              tunnel: [w3009 sgl 0.0] -> w3002
              tunnel: [TRUE ("XScale") FALSE ("XScale")] -> w3006
              tunnel: w2995 -> [w3007 _]
              frame False {
                n367 = local read "Y-lines FreeLine"() -> (w3010:sgl)
                n368 = Subtract(x=w3007, y=w3010) -> (x-y=w3009:sgl)
              }
              frame True {
                n369 = local read "X-pixels FreeLine"() -> (w3014:sgl)
                n370 = local read "Y-lines FreeLine"() -> (w3013:sgl)
              }
            }
            n371 = property on="SlideHorizontal" class="Slide (strict)"("Visible"=w3006) -> ()  [unwired: 2 in, 2 out]
            n372 = property on="SlideHorizontal" class="Slide (strict)"("Scale.Range:Minimum"=0.0, "Scale.Range:Maximum"=w3002) -> ()  [unwired: 2 in, 2 out]
            n373 = Divide(x=w3000, y=w2995) -> (x/y=w3001:sgl)
            n374 = Multiply(x=w2996, y=w2995) -> (x*y=w2999:sgl)
            n375 = Greater?(x=w2999, y=w3000) -> (0:w2998:bool)
            n376 = Select(t=w3001, s=w2998, f=w2996) -> (s? t:f=w2997:sgl)
          }
        }
        n377 = property on="Image 2" class="IntGraph (strict)"() -> ("Color Table"=w2037:u32[])  [unwired: 2 in, 2 out]
        n378 = property on="Histogram1" class="XYGraph (strict)"("Y Scale.Range:Minimum"=w2035, "Y Scale.Range:Maximum"=w2034) -> ()  [unwired: 2 in, 2 out]
        n379 = local read "Fiberscope\nMode"() -> (w1895:bool)
        n380 = Greater Or Equal?(x=w1859, y=u16 3) -> (x >= y?=w1857:bool)
        n381 = property on="Image 3" class="IntGraph (strict)"("X Scale.Range:Minimum"=w2036, "X Scale.Range:Maximum"=w2033, "Y Scale.Range:Minimum"=w2036, "Y Scale.Range:Maximum"=w2032, "Color Table"=w2037) -> ()  [unwired: 2 in, 2 out]
        n382 = property on="Image 4" class="IntGraph (strict)"("X Scale.Range:Minimum"=w2036, "X Scale.Range:Maximum"=w2033, "Y Scale.Range:Minimum"=w2036, "Y Scale.Range:Maximum"=w2032, "Color Table"=w2037) -> ()  [unwired: 2 in, 2 out]
        n383 = property on="Histogram2" class="XYGraph (strict)"("Y Scale.Range:Minimum"=w2035, "Y Scale.Range:Maximum"=w2034) -> ()  [unwired: 2 in, 2 out]
        n384 = local write "Scanpattern"(FALSE ("Scanpattern")) -> ()
        n385 = property on="Histogram1" class="XYGraph (strict)"("X Scale.Range:Minimum"=w2036, "X Scale.Range:Maximum"=w2033) -> ()  [unwired: 2 in, 2 out]
        n386 = property on="Histogram2" class="XYGraph (strict)"("X Scale.Range:Minimum"=w2036, "X Scale.Range:Maximum"=w2033) -> ()  [unwired: 2 in, 2 out]
        n387 = case shown="True" w1857 {
          tunnel: [w2047 w2048] -> w1856
          frame False {
            n388 = local read "pixel dwell time [us]"() -> (w2047:sgl)
          }
          frame True {
            n389 = local read "pixel dwell time [us] FreeLine"() -> (w2048:sgl)
          }
        }
        n390 = local read "Mode selectorFScope"() -> (w1892:u16)
        n391 = local read "#"() -> (w1865:sgl)
        n392 = Array Subset(array=w1868, length (col)=w1865) -> (w1867:u8[][])  [unwired: 3 in]
        n393 = flat-sequence {
          tunnel: [w2986] -> w1922
          frame #0 {
            n394 = call <vilib>:"DAQmx Reset Device.vi"("device in"="AO/DIO Device") -> ("error out"=w2985:errorcluster)  [unwired: 14 in]
            n395 = call <vilib>:"DAQmx Reset Device.vi"("device in"="AI Device", "error in"=w2985) -> ("error out"=w2986:errorcluster)  [unwired: 13 in]
          }
        }
        n396 = local read "AO/DIO Device"() -> (w1942:tag)
        n397 = local read "AO/DIO Device"() -> (w1946:tag)
        n398 = case shown="True" "Test Run?" {
          tunnel: w1867 -> [_ w2049]
          frame False {
          }
          frame True {
            "Image3Arrayd" <- w2049
          }
        }
        n399 = Concatenate Strings(tag "/" ("destination terminal"), w1942, tag "/ao/SampleClock" ("source of ticks")) -> (w1943:string)
        n400 = Concatenate Strings(w1946, tag "/ctr0" ("counter")) -> (w1944:string)
        n401 = Type Cast(type=tag "" ("source of ticks"), x=w1943) -> (*(type *) &x=w1938:tag)
        n402 = Type Cast(type=tag "" ("counter"), x=w1944) -> (*(type *) &x=w1926:tag)
        n403 = local read "frame/line indicator"() -> (w1919:u16)
        n404 = local read "AO/DIO Device"() -> (w2001:tag)
        n405 = case shown="False" w1895 {
          tunnel: w1872 -> [w2106 _]
          tunnel: w1859 -> [w2105 _]
          tunnel: "new FreeLine?" -> [w2104 _]
          tunnel: [w2103 FALSE ("XScale")] -> w1862
          tunnel: [w2102 w2860] -> w2015
          tunnel: [w2101 w2853] -> w2005
          tunnel: [w2100 w2863] -> w1888
          tunnel: w2001 -> [w2099 w2858]
          tunnel: tag "" ("physical channels") -> [w2098 w2859]
          tunnel: [w2097 w2856] -> w1879
          tunnel: [w2096 sgl 1.0 ("total y pixels")] -> w1953
          tunnel: [w2095 w2856] -> w1947
          tunnel: [w2094 w2855] -> w1915
          tunnel: w1892 -> [_ w2854]
          tunnel: w1887 -> [w2093 _]
          tunnel: w1886 -> [w2092 _]
          tunnel: w1873 -> [w2091 _]
          tunnel: w1871 -> [w2090 _]
          tunnel: w1870 -> [w2089 _]
          tunnel: w1864 -> [w2088 _]
          tunnel: w1863 -> [w2087 _]
          tunnel: [w2086 FALSE ("XScale")] -> w1861
          tunnel: [w2085 _] -> w1860
          frame False {
            n406 = case shown="0, Default" w2105 {
              tunnel: w2106 -> [_ _ _ w2596 w2700]
              tunnel: [w2175 w2270 w2469 w2591 w2699] -> w2101
              tunnel: [w2188 w2291 w2461 w2594 w2698] -> w2095
              tunnel: [w2190 w2295 w2463 w2593 w2697] -> w2097
              tunnel: [w2178 w2294 w2464 w2595 w2701] -> w2096
              tunnel: w2104 -> [_ _ _ w2592 w2695]
              tunnel: [w2187 w2270 w2469 w2591 w2699] -> w2100
              tunnel: [FALSE ("XScale") FALSE ("XScale") FALSE ("XScale") FALSE ("XScale") TRUE ("XScale")] -> w2103
              tunnel: [w2173 w2265 w2527 w2584 w2687] -> w2102
              tunnel: w2099 -> [w2111 w2269 w2528 w2586 w2689]
              tunnel: w2098 -> [w2174 w2268 w2529 w2585 w2688]
              tunnel: [w2172 w2293 w2462 w2581 w2685] -> w2094
              tunnel: w2093 -> [_ _ _ _ w2684]
              tunnel: w2092 -> [_ _ _ _ w2683]
              tunnel: w2091 -> [_ w2292 _ _ _]
              tunnel: w2090 -> [w2170 w2355 w2459 w2579 w2682]
              tunnel: w2089 -> [w2169 w2354 w2456 w2580 w2681]
              tunnel: w2088 -> [w2168 w2353 w2522 _ _]
              tunnel: w2087 -> [_ _ _ _ _]
              tunnel: [FALSE ("XScale") FALSE ("XScale") TRUE ("XScale") FALSE ("XScale") FALSE ("XScale")] -> w2086
              tunnel: [w2107 w2276 _ _ _] -> w2085
              frame 0, Default {
                w2171 = 10123 items=["Finite Samples"=10178, "Continuous Samples"=10123, "Hardware Timed Single Point"=12522] ("sample mode")
                n407 = local read "On?"() -> (w2115:bool)
                n408 = local read "[µm] per pixel at zoom 1"() -> (w2120:sgl)
                n409 = local read "Y-lines"() -> (w2119:sgl)
                n410 = local read "Rotation z"() -> (w2114:sgl)
                n411 = case shown="False" w2115 {
                  tunnel: w2114 -> [_ w2237]
                  tunnel: [sgl 0.0 ("Rotation z") w2237] -> w2113
                  frame False {
                  }
                  frame True {
                  }
                }
                n412 = Divide(x=w2113, y=360.0) -> (x/y=w2166:dbl)
                n413 = Multiply(x=w2166, y=6.283185307179586) -> (x*y=w2164:dbl)
                n414 = Build Array(w2170, w2169, w2168) -> (w2150:dbl[][])
                "OriginalScanSignals" <- w2150
                n415 = Sine(x=w2164) -> (sin(x)=w2123:dbl)
                n416 = Cosine(x=w2164) -> (cos(x)=w2163:dbl)
                n417 = Multiply(x=w2120, y=w2119) -> (x*y=w2117:sgl)
                n418 = Negate(x=w2123) -> (-x=w2162:dbl)
                n419 = Array Subset(array=w2150, length (row)=1 ("length")) -> (w2153:dbl[][])  [unwired: 3 in]
                n420 = Array Subset(array=w2150, index (row)=1 ("index")) -> (w2157:dbl[][])  [unwired: 3 in]
                n421 = local read "Zoom"() -> (w2124:sgl)
                n422 = Build Array(w2123, w2163) -> (w2159:dbl[])
                n423 = Build Array(w2163, w2162) -> (w2160:dbl[])
                n424 = local read "total y pixels"() -> (w2178:sgl)
                n425 = Build Array(w2160, w2159) -> (w2158:dbl[][])
                n426 = local read "Rotation"() -> (w2180:sgl)
                n427 = call-poly <vilib>:"A x B.vi"("B"=w2157, "A"=w2158) -> ("A x B"=w2151:T15)  [unwired: 1 out]
                n428 = local read "Position piezo [µm]"() -> (w2122:sgl)
                n429 = Divide(x=w2117, y=w2124) -> (x/y=w2128:sgl)
                n430 = local read "total x pixels"() -> (w2190:sgl)
                n431 = Divide(x=w2128, y=sgl 40.0) -> (x/y=w2134:sgl)
                n432 = Multiply(x=w2180, y=-1.0) -> (x*y=w2183:dbl)
                n433 = Index Array(array=w2151, index (row)=0 ("disabled index (col)")) -> (element=w2152:dbl[])  [unwired: 1 in]
                n434 = Index Array(array=w2151, index (row)=1 ("disabled index (col)")) -> (element=w2125:dbl[])  [unwired: 1 in]
                n435 = Array Max & Min(array=w2125) -> (max value=w2126:dbl, min value=w2131:dbl)  [unwired: 2 out]
                n436 = Subtract(x=w2126, y=w2131) -> (x-y=w2133:dbl)
                n437 = Equal To 0?(x=w2133) -> (x = 0?=w2136:bool)
                n438 = Subtract(x=w2125, y=w2131) -> (x-y=w2137:dbl[])
                n439 = Subtract(x=w2183, y=360.0) -> (x-y=w2181:dbl)
                n440 = local read "FocusModeSelector"() -> (w2110:bool)
                n441 = Multiply(x=w2134, y=w2123) -> (x*y=w2135:dbl)
                n442 = Divide(x=w2181, y=360.0) -> (x/y=w2196:dbl)
                n443 = Build Array (concatenate)(w2153, w2152) -> (w2149:dbl[][])
                n444 = Divide(x=w2122, y=sgl 40.0) -> (x/y=w2118:sgl)
                n445 = case shown="False" w2136 {
                  tunnel: [w2250 w2251] -> w2132
                  tunnel: w2133 -> [w2249 _]
                  tunnel: w2135 -> [w2247 _]
                  tunnel: w2118 -> [w2245 w2253]
                  tunnel: w2137 -> [w2239 w2252]
                  frame False {
                    n446 = Divide(x=w2239, y=w2249) -> (x/y=w2248:dbl[])
                    n447 = Multiply(x=w2248, y=w2247) -> (x*y=w2246:dbl[])
                    n448 = Add(x=w2246, y=w2245) -> (x+y=w2238:dbl[])
                    n449 = Array Max & Min(array=w2238) -> (max value=w2244:dbl, min value=w2241:dbl)  [unwired: 2 out]
                    n450 = Subtract(x=w2244, y=w2241) -> (x-y=w2243:dbl)
                    n451 = Divide(x=w2243, y=2.0) -> (x/y=w2240:dbl)
                    n452 = Subtract(x=w2238, y=w2240) -> (x-y=w2250:dbl[])
                  }
                  frame True {
                    n453 = Add(x=w2252, y=w2253) -> (x+y=w2251:dbl[])
                  }
                }
                n454 = Multiply(x=w2196, y=6.283185307179586) -> (x*y=w2198:dbl)
                n455 = Sine(x=w2198) -> (sin(x)=w2202:dbl)
                n456 = Cosine(x=w2198) -> (cos(x)=w2203:dbl)
                n457 = Negate(x=w2202) -> (-x=w2199:dbl)
                n458 = Not(x=w2110) -> (.not. x?=w2108:bool)
                n459 = Build Array(w2203, w2199) -> (w2200:dbl[])
                n460 = Build Array(w2202, w2203) -> (w2201:dbl[])
                n461 = Build Array(w2200, w2201) -> (w2179:dbl[][])
                n462 = Bundle("sample mode"=w2171, "sample mode"=w2171) -> (w2172:cluster{"sample mode":i32, "sample mode":i32})  [unwired: 1 in]
                n463 = call-poly <vilib>:"A x B.vi"("B"=w2149, "A"=w2179) -> ("A x B"=w2148:T15)  [unwired: 1 out]
                n464 = In Range and Coerce(upper limit=0.0 ("element"), x=w2132, lower limit=10.0 ("element")) -> (coerced(x)=w2145:dbl[])  [unwired: 1 out]
                n465 = Divide(x=w2148, y=w2124) -> (x/y=w2147:T15)
                n466 = Array Size(array=w2145) -> (size(s)=w2144:i32)
                n467 = case shown="False" w2110 {
                  tunnel: w2174 -> [w2227 w2235]
                  tunnel: [w2226 w2234] -> w2173
                  tunnel: w2111 -> [w2225 w2233]
                  frame True {
                    n468 = Concatenate Strings(w2225, tag "/ao0," ("physical channels"), w2225, tag "/ao1," ("physical channels"), w2225, tag "/ao2" ("physical channels")) -> (w2222:string)
                    n469 = Type Cast(type=w2227, x=w2222) -> (*(type *) &x=w2226:tag)
                  }
                  frame False {
                    n470 = Concatenate Strings(w2233, tag "/ao0," ("physical channels"), w2233, tag "/ao1," ("physical channels"), w2233, tag "/ao2," ("physical channels"), w2233, tag "/ao3" ("physical channels")) -> (w2230:string)
                    n471 = Type Cast(type=w2235, x=w2230) -> (*(type *) &x=w2234:tag)
                  }
                }
                n472 = Index Array(array=w2147, index (row)=0 ("disabled index (col)")) -> (element=w2194:dbl[])  [unwired: 1 in]
                n473 = Index Array(array=w2147, index (row)=1 ("disabled index (col)")) -> (element=w2193:dbl[])  [unwired: 1 in]
                n474 = Multiply(x=w2144, y=15) -> (x*y=w2139:i32)
                n475 = Divide(x=w2139, y=360.0) -> (x/y=w2140:dbl)
                n476 = Add(x=w2193, y="y jog") -> (x+y=w2185:dbl[])
